vi "app_pktRebuild.vi"(8 "reset":bool=TRUE, 11 "app_pkt":T1(array[cluster])) -> (3 "out pkts":string[](array[string]))   [LabVIEW 2014]
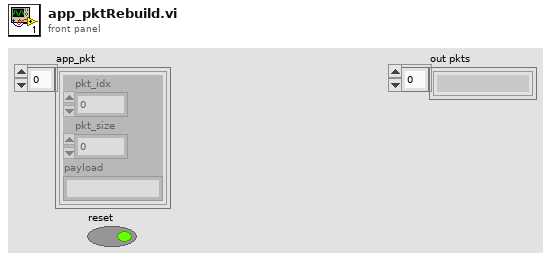
[diagram p1: front panel]
types:
  T1 = cluster{"pkt_idx":u32, "pkt_size":u32, "payload":string}[]
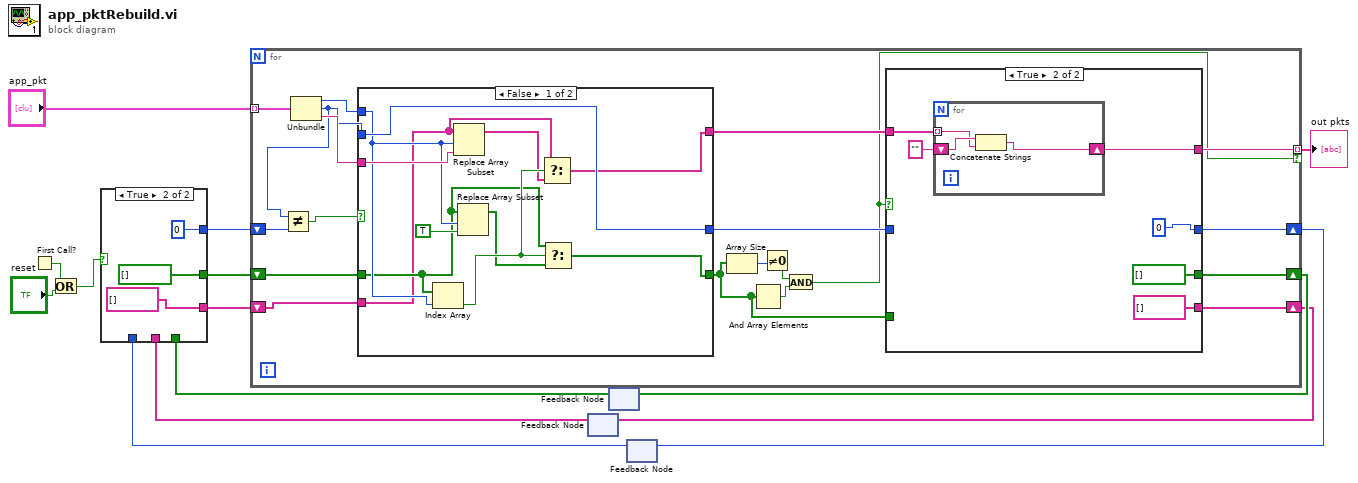
[diagram p0: block diagram]
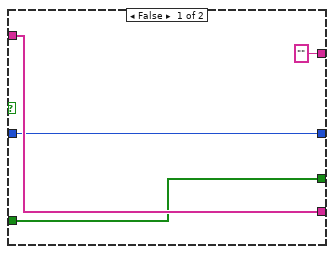
[diagram p3: hidden frame]
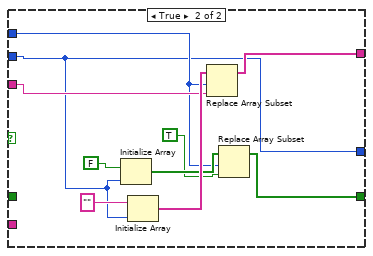
[diagram p4: hidden frame]
diagram:
  n1 = First Call?() -> (First Call?: T/F=w10:bool)
  n2 = Or(x=w10, y="reset") -> (x .or. y?=w8:bool)
  n3 = feedback #1() -> (w4:string[])  [unwired: 1 in]
  n4 = feedback #2() -> (w6:bool[])  [unwired: 1 in]
  n5 = feedback #3() -> (w2:u32)  [unwired: 1 in]
  n6 = case shown="True" w8 {
    tunnel: [w17 u32 0] -> w13
    tunnel: [w16 bool[] []] -> w12
    tunnel: [w15 string[] []] -> w11
    tunnel: w6 -> [w16 _]
    tunnel: w4 -> [w15 _]
    tunnel: w2 -> [w17 _]
    frame False {
    }
    frame True {
    }
  }
  n7 = for {
    tunnel: "app_pkt" -> [w39] mode=indexing
    shift-right: [w24] -> w3
    shift-left: w13 -> [w38]
    shift-right: [w23] -> w7
    shift-left: w12 -> [w36]
    shift-right: [w25] -> w5
    shift-left: w11 -> [w35]
    tunnel: [w22] -> w1 mode=indexing if=w21
    n8 = Unbundle(w39) -> ("pkt_idx"=w34:u32, "pkt_size"=w32:u32, "payload"=w33:string)
    n9 = Not Equal?(x=w32, y=w38) -> (x != y?=w37:bool)
    n10 = case shown="False" w37 {
      tunnel: w36 -> [w56 _]
      tunnel: w35 -> [w55 _]
      tunnel: w34 -> [w60 w68]
      tunnel: w32 -> [w61 w64]
      tunnel: w33 -> [w63 w71]
      tunnel: [w54 w65] -> w26
      tunnel: [w53 w66] -> w28
      tunnel: [w61 w64] -> w27
      frame False {
        n11 = Index Array(array=w56, index=w60) -> (element=w59:bool)
        n12 = Replace Array Subset(array=w55, new element=w63, index=w60) -> (w58:string[])
        n13 = Replace Array Subset(array=w56, new element=TRUE, index=w60) -> (w57:bool[])
        n14 = Select(t=w55, s=w59, f=w58) -> (s? t:f=w54:string[])
        n15 = Select(t=w56, s=w59, f=w57) -> (s? t:f=w53:bool[])
      }
      frame True {
        n16 = Initialize Array(FALSE, w64) -> (w69:bool[])
        n17 = Initialize Array("", w64) -> (w72:string[])
        n18 = Replace Array Subset(array=w72, new element=w71, index=w68) -> (w65:string[])
        n19 = Replace Array Subset(array=w69, new element=TRUE, index=w68) -> (w66:bool[])
      }
    }
    n20 = Array Size(array=w28) -> (size(s)=w31:i32)
    n21 = And Array Elements(Boolean array=w28) -> (logical AND=w29:bool)
    n22 = Not Equal To 0?(x=w31) -> (x != 0?=w30:bool)
    n23 = And(x=w30, y=w29) -> (x .and. y?=w21:bool)
    n24 = case shown="True" w21 {
      tunnel: w28 -> [w41 _]
      tunnel: w27 -> [w42 _]
      tunnel: w26 -> [w43 w46]
      tunnel: [w43 string[] []] -> w25
      tunnel: [w42 0] -> w24
      tunnel: [w41 bool[] []] -> w23
      tunnel: ["" w44] -> w22
      frame False {
      }
      frame True {
        n25 = for {
          tunnel: w46 -> [w51] mode=indexing
          shift-right: [w50] -> w44
          shift-left: "" -> [w52]
          n26 = Concatenate Strings(w52, w51) -> (w50:string)
        }
      }
    }
  }
  "out pkts" <- w1
  n27 = feedback-in #1(w5) -> ()
  n28 = feedback-in #2(w7) -> ()
  n29 = feedback-in #3(w3) -> ()
